vi "Delete waveform file.vi"(7 "File IO parameters":T1={"Output Folder"=path "C:/Users/Abigail/Documents/Imperial Optical software/Optical Software Code Simplified/Output", "Error file"=path "Error Log.txt", "Config file"=path "Config.ini", "File prefix"="", "Waveform read"={"t0"=timestamp(0 s since 1904-01-01), "dt"=1.0, "Y"=[]}}, 8 "error in":errorcluster, 11 "Dataset name":string="DAQ (raw data)") -> (0 "error out":errorcluster)   [LabVIEW 2017, in "File IO.lvlib"]
uses:
  File IO.lvlib
  Controls/Params.ctl
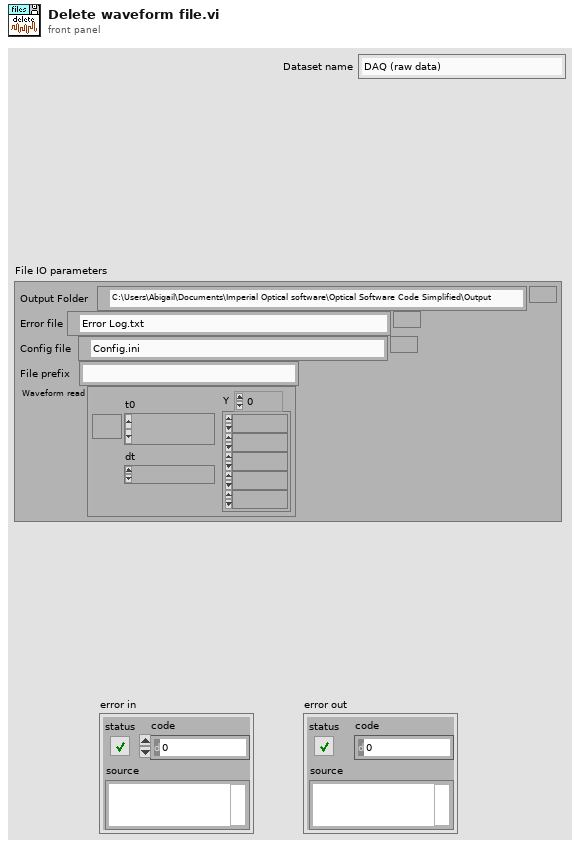
[diagram p1: front panel]
types:
  T1 = typedef "File IO.lvlib/Params.ctl" = cluster{"Output Folder":path, "Error file":path, "Config file":path, "File prefix":string, "Waveform read":waveform(dbl)}
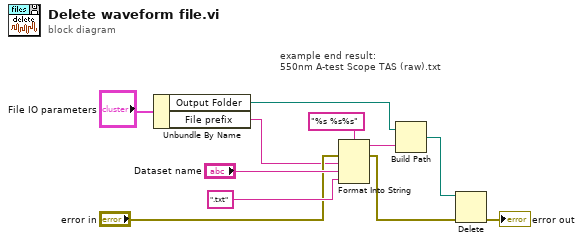
[diagram p0: block diagram]
diagram:
  # "example end result:\n550nm A-test Scope TAS (raw).txt"
  n1 = Unbundle By Name("File IO parameters") -> ("Output Folder"=w11:path, "File prefix"=w3:string)
  n2 = Format Into String(format string="%s %s%s", error in="error in", w3, "Dataset name", ".txt" ("Dataset name 2")) -> (resulting string=w7:string, error out=w4:errorcluster)  [unwired: 1 in]
  n3 = Build Path(base path=w11, name or relative path=w7) -> (appended path=w2:path)
  n4 = Delete(path (use dialog)=w2, error in=w4) -> (error out=→"error out":errorcluster)  [unwired: 3 in, 2 out]
